vi "kalmanCheckData.vi"(0 "x_k":T1, 1 "Pk":T1, 2 "R":T1, 4 "Variance Memory":i32=1, 5 "error in (no error)":errorcluster) -> (14 "x_k out":T1, 15 "Pk out":T1, 16 "R out":T1, 19 "error out":errorcluster)   [LabVIEW 2023, in "Vision.lvclass"]
uses:
  Vision.lvclass
  <vilib>/Analysis/Matrix/Datatypes/RealMatrix.ctl
  <vilib>/Analysis/Matrix/Numeric/Conversions/Array To Matrix - RA2.vi
  <vilib>/Analysis/7linalg.llb/Create Special Real Matrix.vi
  <vilib>/Analysis/Matrix/NI_Matrix.lvlib
  <vilib>/Analysis/NI_AALPro.lvlib
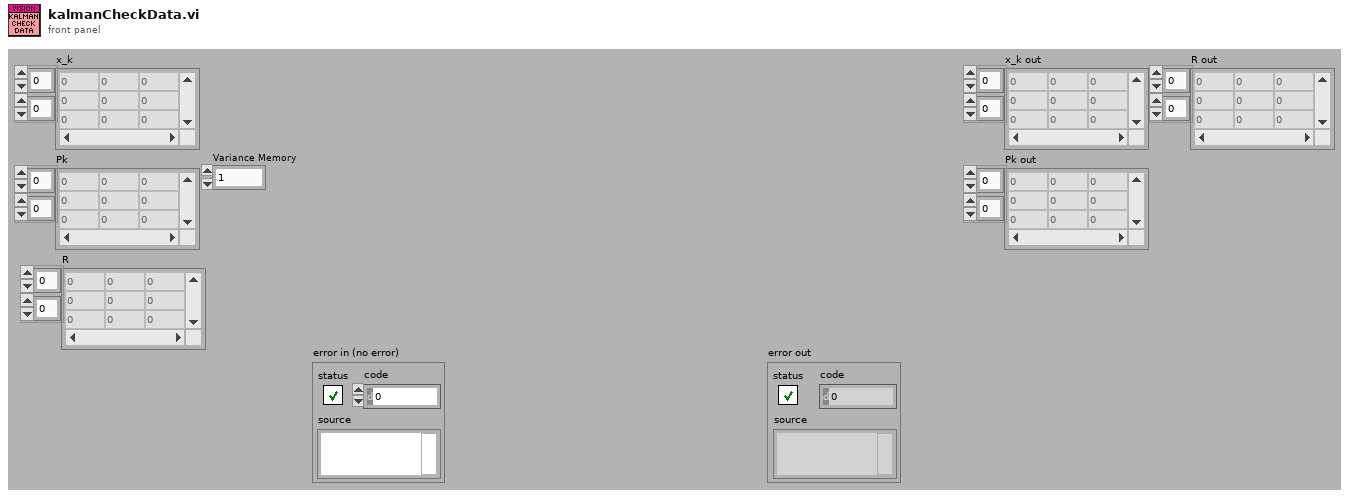
[diagram p1: front panel]
types:
  T1 = typedef "NI_Matrix.lvlib/RealMatrix.ctl" = dbl[][]
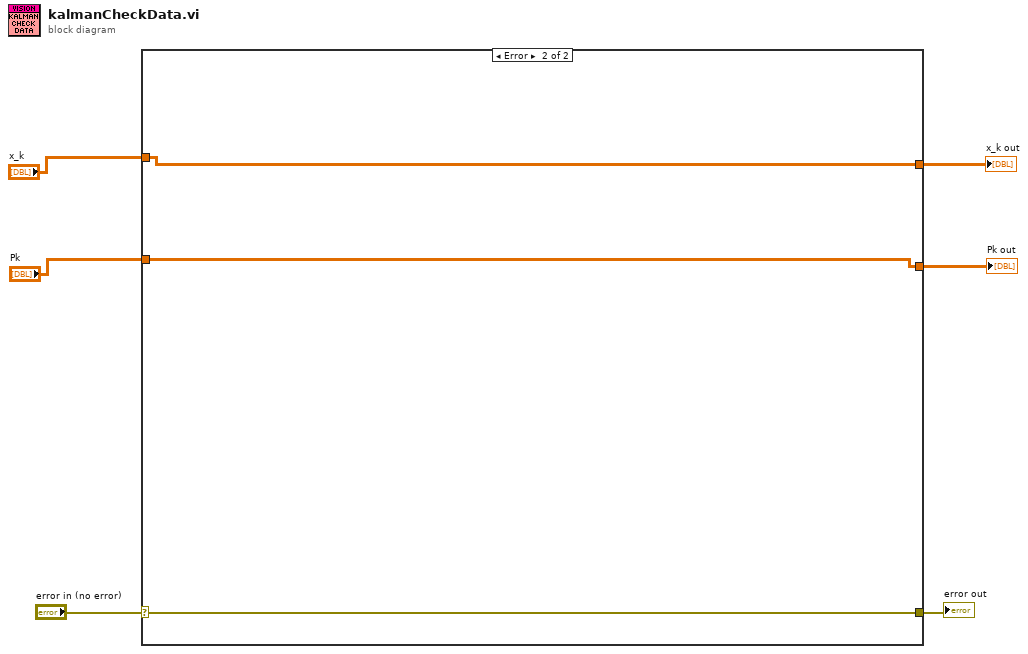
[diagram p0: block diagram]
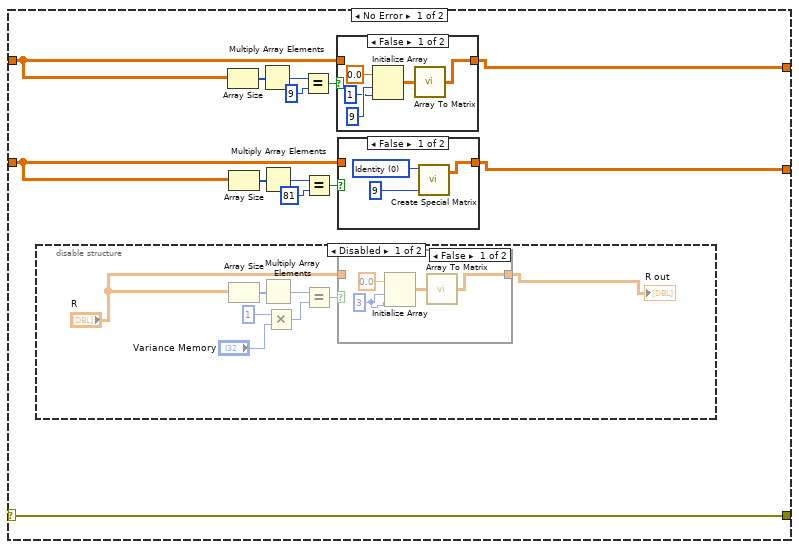
[diagram p2: hidden frame]
diagram:
  n1 = case shown="Error" "error in (no error)" {
    selector: "error in (no error)" -> [w19 w45]
    tunnel: [w19 w45] -> w5
    tunnel: "Pk" -> [w10 w43]
    tunnel: "x_k" -> [w9 w44]
    tunnel: [w8 w43] -> w2
    tunnel: [w7 w44] -> w1
    frame No Error {
      n2 = disable-structure shown="Disabled" {
        frame Disabled {
          n3 = Array Size(array="R") -> (size(s)=w25:i32[])
          n4 = Multiply Array Elements(1:w25) -> (0:w26:i32)
          n5 = Multiply(x=1, y="Variance Memory") -> (x*y=w24:i32)
          n6 = Equal?(x=w26, y=w24) -> (x = y?=w27:bool)
          n7 = case shown="False" w27 {
            tunnel: "R" -> [_ w32]
            tunnel: [w29 w32] -> w21
            frame False {
              w28 = 3 ("dimension size")
              n8 = Initialize Array(0.0 ("element"), w28, w28) -> (w30:dbl[][])
              n9 = call-poly <vilib>:"Array To Matrix.vi"("Real 2D Array"=w30) -> ("Real Matrix"=w29:T1)
            }
            frame True {
            }
          }
          "R out" <- w21
        }
        frame Enabled {
        }
      }
      n10 = Array Size(array=w9) -> (size(s)=w15:i32[])
      n11 = Array Size(array=w10) -> (size(s)=w11:i32[])
      n12 = Multiply Array Elements(1:w15) -> (0:w16:i32)
      n13 = Multiply Array Elements(1:w11) -> (0:w12:i32)
      n14 = Equal?(x=w16, y=9) -> (x = y?=w18:bool)
      n15 = Equal?(x=w12, y=81) -> (x = y?=w14:bool)
      n16 = case shown="False" w18 {
        tunnel: w9 -> [_ w42]
        tunnel: [w38 w42] -> w7
        frame False {
          n17 = Initialize Array(0.0 ("element"), 9 ("dimension size"), 1 ("dimension size")) -> (w39:dbl[][])
          n18 = call-poly <vilib>:"Array To Matrix.vi"("Real 2D Array"=w39) -> ("Real Matrix"=w38:T1)
        }
        frame True {
        }
      }
      n19 = case shown="False" w14 {
        tunnel: w10 -> [_ w36]
        tunnel: [w33 w36] -> w8
        frame False {
          w35 = 0 items=["Identity", "Diagonal", "Toeplitz", "Vandermonde", "Companion", "Hankel", "Hadamard", "Wilkinson", "Hilbert", "Inverse Hilbert", "Rosser", "Pascal"] ("matrix type")
          n20 = call-poly <vilib>:"Create Special Matrix.vi"("matrix type"=w35, "matrix size"=9) -> ("Special Matrix"=w33:T1)  [unwired: 3 in, 1 out]
        }
        frame True {
        }
      }
    }
    frame Error {
    }
  }
  "error out" <- w5
  "x_k out" <- w1
  "Pk out" <- w2
